vi "Flash_Sample.vi"() -> ()   [LabVIEW 2020]
uses:
  Lib/JLinkARM.lvlib
panel:
  in  "Erase":bool
  in  "Prog. addr. (bin file only)":u32 format="0x%08x"
  in  "Data File":path
  in  "Program":bool
  in  "Interface":string(combo)
  out "Error":bool
  out "Busy":bool
  out "Success":bool
  in  "Exit":bool
  in  "TIF Speed [kHz]:":dbl
  in  "Device:":string
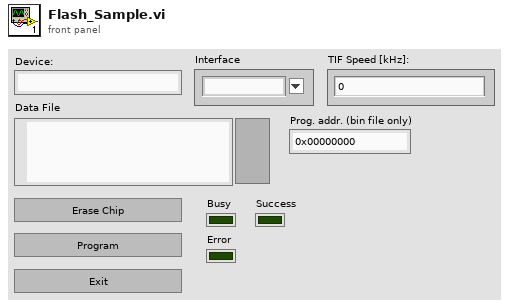
[diagram p1: front panel]
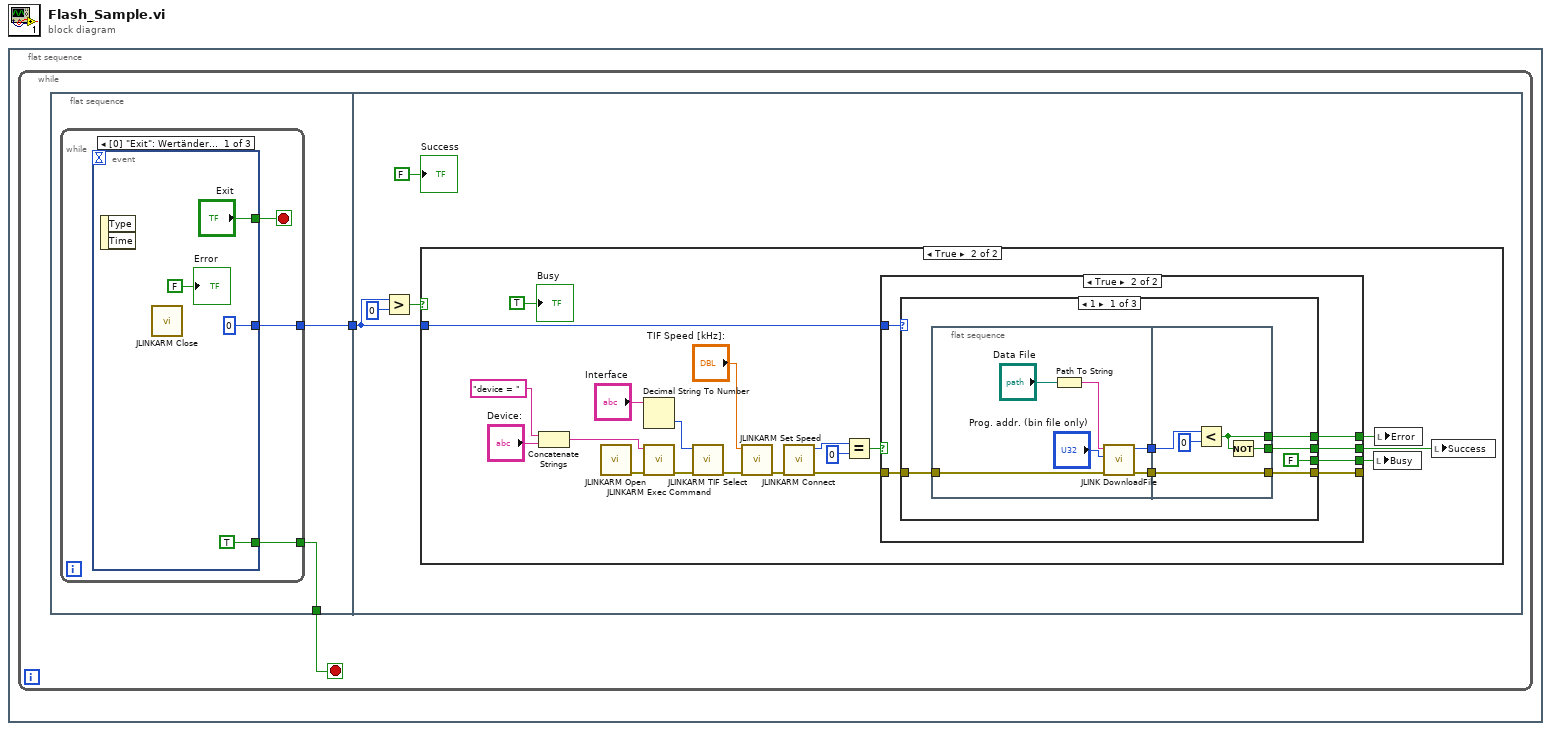
[diagram p0: block diagram]
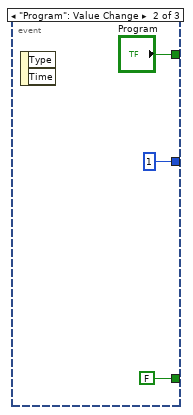
[diagram p2: hidden frame]
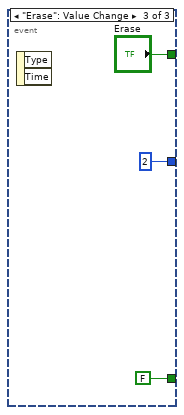
[diagram p3: hidden frame]
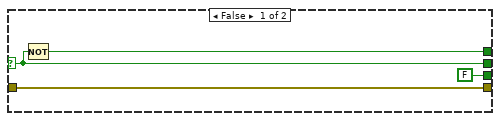
[diagram p5: hidden frame]
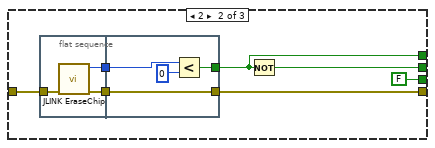
[diagram p6: hidden frame]
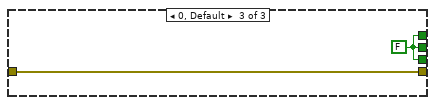
[diagram p7: hidden frame]
diagram:
  n1 = flat-sequence {
    frame #0 {
      n2 = while {
        stop <- w1 stop-if-true
        n3 = flat-sequence {
          tunnel: [w4] -> w2
          tunnel: [w3] -> w1
          tunnel: w2 -> [w20]
          frame #0 {
            n4 = while {
              tunnel: [w6] -> w4
              tunnel: [w5] -> w3
              stop <- w7 stop-if-true
              n5 = event shown="[0] \"Exit\": Wertänderung" {
                selector: _ -> [_ _ _]
                dyn-events: _ -> [_ _ _]
                timeout: _ -> [_ _ _]
                tunnel: ["Exit" "Program" "Erase"] -> w7
                tunnel: [0 1 2] -> w6
                tunnel: [TRUE FALSE FALSE] -> w5
                event "Exit": Value Change {
                  n6 = event-data() -> ()  [unwired: 1 in, 2 out]
                  n7 = call "JLINKARM Close.vi"() -> ()  [unwired: 11 in, 1 out]
                  "Error" <- FALSE
                }
                event "Program": Value Change {
                  n8 = event-data() -> ()  [unwired: 1 in, 2 out]
                }
                event "Erase": Value Change {
                  n9 = event-data() -> ()  [unwired: 1 in, 2 out]
                }
              }
            }
          }
          frame #1 {
            n10 = Greater?(x=w20, y=0) -> (0:w19:bool)
            n11 = case shown="True" w19 {
              tunnel: w20 -> [_ w28]
              frame False {
              }
              frame True {
                n12 = Concatenate Strings("device = ", "Device:") -> (w32:string)
                n13 = call "JLINKARM Open.vi"() -> ("error out"=w36:errorcluster)  [unwired: 10 in, 1 out]
                n14 = Decimal String To Number(string="Interface") -> (number=w31:i32)  [unwired: 2 in, 1 out]
                n15 = call "JLINKARM Exec Command.vi"("error in (no error)"=w36, "pIn"=w32) -> ("error out"=w35:errorcluster)  [unwired: 7 in, 2 out]
                n16 = call "JLINKARM TIF Select.vi"("error in (no error)"=w35, "Interface"=w31) -> ("error out"=w34:errorcluster)  [unwired: 8 in, 1 out]
                n17 = call "JLINKARM Set Speed.vi"("error in (no error)"=w34, "Speed"="TIF Speed [kHz]:") -> ("error out"=w33:errorcluster)  [unwired: 9 in]
                n18 = call "JLINKARM Connect.vi"("error in (no error)"=w33) -> ("error out"=w27:errorcluster, "function return"=w29:i32)  [unwired: 9 in]
                n19 = Equal?(x=w29, y=0) -> (x = y?=w23:bool)
                n20 = case shown="True" w23 {
                  selector: w23 -> [w43 _]
                  tunnel: w28 -> [_ w50]
                  tunnel: w27 -> [w42 w49]
                  tunnel: [w44 w48] -> w25
                  tunnel: [w43 w47] -> w24
                  tunnel: [w42 w46] -> _
                  tunnel: [FALSE w45] -> w22
                  frame False {
                    n21 = Not(x=w43) -> (.not. x?=w44:bool)
                  }
                  frame True {
                    n22 = case shown="1" w50 {
                      tunnel: w49 -> [w57 w75 w84]
                      tunnel: [w54 w71 w83] -> w48
                      tunnel: [w53 w72 w83] -> w47
                      tunnel: [w52 w70 w84] -> w46
                      tunnel: [FALSE FALSE w83] -> w45
                      frame 1 {
                        n23 = flat-sequence {
                          tunnel: w57 -> [w63]
                          tunnel: [w59] -> w56
                          tunnel: [w58] -> w55
                          tunnel: w56 -> [w67]
                          tunnel: w55 -> [w68]
                          tunnel: [w68] -> w52
                          tunnel: [w65] -> w53
                          tunnel: [w64] -> w54
                          frame #0 {
                            n24 = Path To String(path="Data File") -> (string=w60:string)
                            n25 = call "JLINK DownloadFile.vi"("error in (no error)"=w63, "Prog. addr. (bin file only)"="Prog. addr. (bin file only)", "File Path"=w60) -> ("error out"=w58:errorcluster, "Return value"=w59:i32)  [unwired: 7 in]
                          }
                          frame #1 {
                            n26 = Less?(x=w67, y=0) -> (x < y?=w64:bool)
                            n27 = Not(x=w64) -> (.not. x?=w65:bool)
                          }
                        }
                      }
                      frame 2 {
                        n28 = flat-sequence {
                          tunnel: w75 -> [w78]
                          tunnel: [w77] -> w74
                          tunnel: [w76] -> w73
                          tunnel: [w82] -> w70
                          tunnel: w74 -> [w82]
                          tunnel: w73 -> [w80]
                          tunnel: [w79] -> w71
                          frame #0 {
                            n29 = call "JLINK EraseChip.vi"("error in (no error)"=w78) -> ("error out"=w77:errorcluster, "Return value"=w76:i32)  [unwired: 9 in]
                          }
                          frame #1 {
                            n30 = Less?(x=w80, y=0) -> (x < y?=w79:bool)
                          }
                        }
                        n31 = Not(x=w71) -> (.not. x?=w72:bool)
                      }
                      frame 0, Default {
                        w83 = FALSE
                      }
                    }
                  }
                }
                n32 = local write "Busy"(w22) -> ()
                n33 = local write "Error"(w25) -> ()
                n34 = local write "Success"(w24) -> ()
                "Busy" <- TRUE
              }
            }
            "Success" <- FALSE
          }
        }
      }
    }
  }
